vi "tmp_unchecked.vi"() -> ()   [LabVIEW 2014]
panel:
  in  "Change/update":dbl
  out "Current Speed":dbl
  in  "MS/update":u32
  in  "Desired Speed":dbl
  # "Always have DS divisible by C/u!"
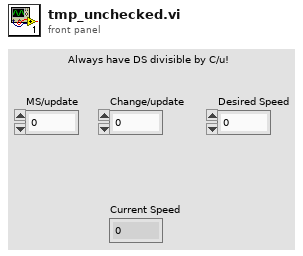
[diagram p1: front panel]
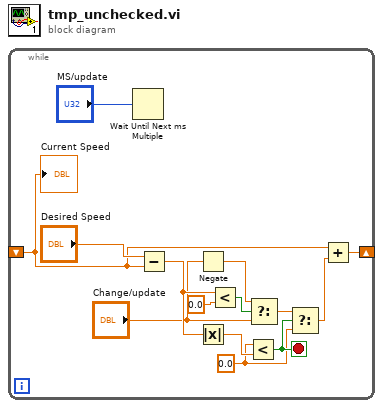
[diagram p0: block diagram]
diagram:
  n1 = while {
    shift-right: [w10] -> _
    shift-left: _ -> [w9]
    stop <- w5 stop-if-true
    w3 = 0.0 ("f")
    n2 = Wait Until Next ms Multiple(millisecond multiple="MS/update") -> ()  [unwired: 1 out]
    n3 = Subtract(x="Desired Speed", y=w9) -> (x-y=w6:dbl)
    n4 = Negate(x="Change/update") -> (-x=w1:dbl)
    n5 = Absolute Value(x=w6) -> (abs(x)=w4:dbl)
    n6 = Less?(x=w6, y=0.0) -> (x < y?=w11:bool)
    n7 = Less?(x=w3, y=w4) -> (x < y?=w5:bool)
    n8 = Select(t=w1, s=w11, f="Change/update") -> (s? t:f=w7:dbl)
    n9 = Select(t=w7, s=w5, f=w3) -> (s? t:f=w8:dbl)
    n10 = Add(x=w9, y=w8) -> (x+y=w10:dbl)
    "Current Speed" <- w9
  }
